vi "MOKE_Teperature and FIeld Sweep_1022D.vi"() -> ()   [LabVIEW 2022 SP3]
uses:
  <vilib>/Analysis/baseanly.llb/Mean (DBL).vi
  <vilib>/Utility/file.llb/Write Delimited Spreadsheet (string).vi
  <vilib>/Utility/file.llb/Write Delimited Spreadsheet (DBL).vi
  <vilib>/Analysis/NI_AALBase.lvlib
panel:
  in  "B field Drift Correction":bool
  in  "Scanner2 Drift Range (V)":dbl
  in  "Scanner1 Drift Range (V)":dbl
  in  "ANC300 address":refnum<visa-resource-name>="COM8"
  in  "Num Averages":i32=100
  in  "Read Status":bool
  in  "Wait for position/focus check every (Oe)":i32
  out "Rh1 B/A v F":cluster{dbl[], dbl[]}(graph)
  out "Temperature Status":i32(ring) items=["TemperatureUnknown"=0, "Stable"=1, "Tracking"=2, "Near"=5, "Chasing"=6, "Filling"=7, "Standby"=10, "Disabled"=13, "ImpedanceNotFunction"=14, "TempFailure"=15]
  out "Field Status":i32(ring) items=["MagnetUnknown"=0, "StablePersistent"=1, "WarmingSwitch"=2, "CoolingSwitch"=3, "StableDriven"=4, "Iterating"=5, "Charging"=6, "Discharging"=7, "CurrentError"=8, "MagnetFailure"=15]
  out "Field":dbl
  out "Temperature":dbl
  in  "Initialize":bool
  in  "System Stablization (s)":dbl=0.1 format="%#_13g"
  in  "Low Value (Oe)":dbl=-30000.0
  in  "High Value (Oe)":dbl=30000.0
  in  "Sweep Field Approach":i32(ring) items=["Linear", "NoOvershoot", "Oscillate"]
  in  "Sweep F Rate (Oe/s)":dbl=200.0 format="%#_13g"
  in  "Sweep F mode":i32(ring) items=["Persistent", "Driven"]
  in  "Set Fixed T":dbl=2.0
  in  "Fixed Temperature Approach":i32(ring)=1 items=["FastSettle", "NoOvershoot"]
  in  "FIxed T  Rate (K/min)":dbl=20.0
  out "PhaseA-F":cluster{dbl[], dbl[]}(graph)
  out "RA-F":cluster{dbl[], dbl[]}(graph)
  out "Phaseh1B-F":cluster{dbl[], dbl[]}(graph)
  out "Rh1B-F":cluster{dbl[], dbl[]}(graph)
  out "phase B 2":dbl
  in  "Phase B 2":u16(ring)=3 items=["X", "Y", "R", "Theta", "Frequency", "Noise", "Xh1", "Yh1", "Rh1", "Theta h1", "Xh2", "Yh2", "Rh2", "Theta h2"]
  out "phase A 2":dbl
  in  "Phase A 2":u16(ring)=3 items=["X", "Y", "R", "Theta", "Frequency", "Noise", "Xh1", "Yh1", "Rh1", "Theta h1", "Xh2", "Yh2", "Rh2", "Theta h2"]
  out "para1 Measurement (mV) 2":dbl=1.49013e-07
  in  "F Clear Plot A":bool
  in  "Parameter A 2":u16(ring)=2 items=["X", "Y", "R", "Theta", "Frequency", "Noise", "Xh1", "Yh1", "Rh1", "Theta h1", "Xh2", "Yh2", "Rh2", "Theta h2"]
  out "para2 Measurement (uV) 2":dbl=1.49013e-07
  in  "F Clear Plot B":bool
  in  "Parameter B 2":u16(ring)=2 items=["X", "Y", "R", "Theta", "Frequency", "Noise", "Xh1", "Yh1", "Rh1", "Theta h1", "Xh2", "Yh2", "Rh2", "Theta h2"]
  out "Field Setting":dbl format="%#_13g"
  out "Fixed Temperature":dbl
  out "Measured Field":dbl
  out "Field Status":i32(ring) items=["MagnetUnknown"=0, "StablePersistent"=1, "WarmingSwitch"=2, "CoolingSwitch"=3, "StableDriven"=4, "Iterating"=5, "Charging"=6, "Discharging"=7, "CurrentError"=8, "MagnetFailure"=15]
  out "Temperature Status":i32(ring) items=["TemperatureUnknown"=0, "Stable"=1, "Tracking"=2, "Near"=5, "Chasing"=6, "Filling"=7, "Standby"=10, "Disabled"=13, "ImpedanceNotFunction"=14, "TempFailure"=15]
  out "Measuring F":bool
  in  "Step(Oe)":i32=2000
  out "F loop run":i32
  out "Temperature Status":i32(ring) items=["TemperatureUnknown"=0, "Stable"=1, "Tracking"=2, "Near"=5, "Chasing"=6, "Filling"=7, "Standby"=10, "Disabled"=13, "ImpedanceNotFunction"=14, "TempFailure"=15]
  out "Field Status":i32(ring) items=["MagnetUnknown"=0, "StablePersistent"=1, "WarmingSwitch"=2, "CoolingSwitch"=3, "StableDriven"=4, "Iterating"=5, "Charging"=6, "Discharging"=7, "CurrentError"=8, "MagnetFailure"=15]
  out "Fixed Field":dbl
  out "Measured Temperature":dbl
  in  "Delay(T/F)":dbl=5.0
  in  "Set FIxed F (Oe)":dbl format="%#_13g"
  in  "Fixed Field Approach":i32(ring) items=["Linear", "NoOvershoot", "Oscillate"]
  in  "FIxed F Rate (Oe/s)":dbl=100.0 format="%#_13g"
  in  "Fixed F mode":i32(ring) items=["Persistent", "Driven"]
  in  "Sweep Temperature Approach":i32(ring)=1 items=["FastSettle", "NoOvershoot"]
  in  "Sweep T  Rate (K/min)":dbl=10.0
  in  "Sweep T/F":bool
  in  "Remote":bool=TRUE
  in  "IP Address":string="169.254.170.239"
  out "Measuring T":bool
  in  "A Sine Output Amplitude (V)":sgl=0.1
  in  "path (folder + filename)":string="C:\\Users\\Public\\OneDrive\\Desktop\\MOKE program\\sweep files"
  in  "LOCKIN address":refnum<visa-resource-name>="COM3"
  out "PhaseA-T":cluster{dbl[], dbl[]}(graph)
  out "RA-T":cluster{dbl[], dbl[]}(graph)
  out "Phaseh1-T":cluster{dbl[], dbl[]}(graph)
  out "Rh1B-T":cluster{dbl[], dbl[]}(graph)
  out "phase B":dbl
  in  "Phase B":u16(ring)=9 items=["X", "Y", "R", "Theta", "Frequency", "Noise", "Xh1", "Yh1", "Rh1", "Theta h1", "Xh2", "Yh2", "Rh2", "Theta h2"]
  out "phase A":dbl
  in  "Phase A":u16(ring)=3 items=["X", "Y", "R", "Theta", "Frequency", "Noise", "Xh1", "Yh1", "Rh1", "Theta h1", "Xh2", "Yh2", "Rh2", "Theta h2"]
  out "para1 Measurement (mV)":dbl=1.49013e-07
  in  "T Clear Plot A":bool
  in  "Parameter A":u16(ring)=2 items=["X", "Y", "R", "Theta", "Frequency", "Noise", "Xh1", "Yh1", "Rh1", "Theta h1", "Xh2", "Yh2", "Rh2", "Theta h2"]
  out "para2 Measurement (uV)":dbl=1.49013e-07
  in  "T Clear Plot B":bool
  in  "Parameter B":u16(ring)=8 items=["X", "Y", "R", "Theta", "Frequency", "Noise", "Xh1", "Yh1", "Rh1", "Theta h1", "Xh2", "Yh2", "Rh2", "Theta h2"]
  out "Temperature Setting":dbl format="%#_13g"
  in  "Save data or not":bool=TRUE
  in  "Step(K)":i32=10
  out "T loop run":i32
  in  "B frequency":dbl=267.7 format="%#_13g"
  in  "B Input Connection (0: Single-Ended)":u16(ring)=1 items=["Single-Ended Voltage", "Differential Voltage", "1 MOhm Current Gain", "100 MOhm Current Gain"]
  in  "B harmonic 1":u8=2
  in  "B harmonic 2":u8=3
  in  "B reference Manual Phase":dbl=-59.75
  in  "auto phase B":bool=TRUE
  in  "B Sample time (s)":dbl=0.001 min=0.001 max=100.0 step=0.001
  in  "B Sensitivity":u16(ring)=20 items=["1 nV/fA", "2 nV/fA", "5 nV/fA", "10 nV/fA", "20 nV/fA", "50 nV/fA", "100 nV/fA", "200 nV/fA", "500 nV/fA", "1 uV/pA", "2 uV/pA", "5 uV/pA", "10 uV/pA", "20 uV/pA", "50 uV/pA", "100 uV/pA", "200 uV/pA", "500 uV/pA", "1 mV/nA", "2 mV/nA", "5 mV/nA", "10 mV/nA", "20 mV/nA", "50 mV/nA", "100 mV/nA", "200 mV/nA", "500 mV/nA", "1 V/uA"]
  in  "Enable Sync Filter B (open when f<200Hz)":bool
  in  "B Time Constant":u8(ring)=9 items=["10 us", "30 us", "100 us", "300 us", "1 ms", "3 ms", "10 ms", "30 ms", "100 ms", "300 ms", "1 s", "3 s", "10 s", "30 s", "100 s", "300 s", "1 ks", "3 ks"]
  in  "B Reference Source":u8(ring) items=["External", "Internal", "Internal Sweep", "Channel-A"]
  in  "B Low Pass Filter Slope":u8(ring)=2 items=["6 dB/oct", "12 dB/oct", "18 db/oct", "24 dB/oct"]
  in  "A frequency":dbl=267.7 format="%#_13g"
  in  "A Input Connection (0: Single-Ended)":u16(ring)=1 items=["Single-Ended Voltage", "Differential Voltage", "1 MOhm Current Gain", "100 MOhm Current Gain"]
  in  "A harmonic 1":u8=2
  in  "A harmonic 2":u8=3
  in  "A reference Manual Phase":dbl=-59.75
  in  "auto phase A":bool=TRUE
  in  "A Reference Source":u8(ring) items=["External", "Internal", "Internal Sweep"]
  in  "A Sample time (s)":dbl=0.001 min=0.001 max=100.0 step=0.001
  in  "A Time Constant":u8(ring)=9 items=["10 us", "30 us", "100 us", "300 us", "1 ms", "3 ms", "10 ms", "30 ms", "100 ms", "300 ms", "1 s", "3 s", "10 s", "30 s", "100 s", "300 s", "1 ks", "3 ks"]
  in  "Enable Sync Filter A (open when f<200Hz)":bool
  in  "A Sensitivity":u16(ring)=20 items=["1 nV/fA", "2 nV/fA", "5 nV/fA", "10 nV/fA", "20 nV/fA", "50 nV/fA", "100 nV/fA", "200 nV/fA", "500 nV/fA", "1 uV/pA", "2 uV/pA", "5 uV/pA", "10 uV/pA", "20 uV/pA", "50 uV/pA", "100 uV/pA", "200 uV/pA", "500 uV/pA", "1 mV/nA", "2 mV/nA", "5 mV/nA", "10 mV/nA", "20 mV/nA", "50 mV/nA", "100 mV/nA", "200 mV/nA", "500 mV/nA", "1 V/uA"]
  in  "A Low Pass Filter Slope":u8(ring)=2 items=["6 dB/oct", "12 dB/oct", "18 db/oct", "24 dB/oct"]
  in  "stabilization(S)":dbl=0.1 format="%#_13g"
  in  "High Value (K)":dbl=300.0
  in  "Low Value (K)":dbl=2.0
  in  "loop #":i32=1
  # "Status"
  # "opticool ip addresse: 169.254.170.239"
  # "Lock-in Setting"
  # "Channel A"
  # "Channel B"
  # "Sweep F Mesurement"
  # "Temprature and Field Setting"
  # "Sweep T Mesurement"
  # "Sweep F"
  # "Sweep T"
  # "0 for no checks"
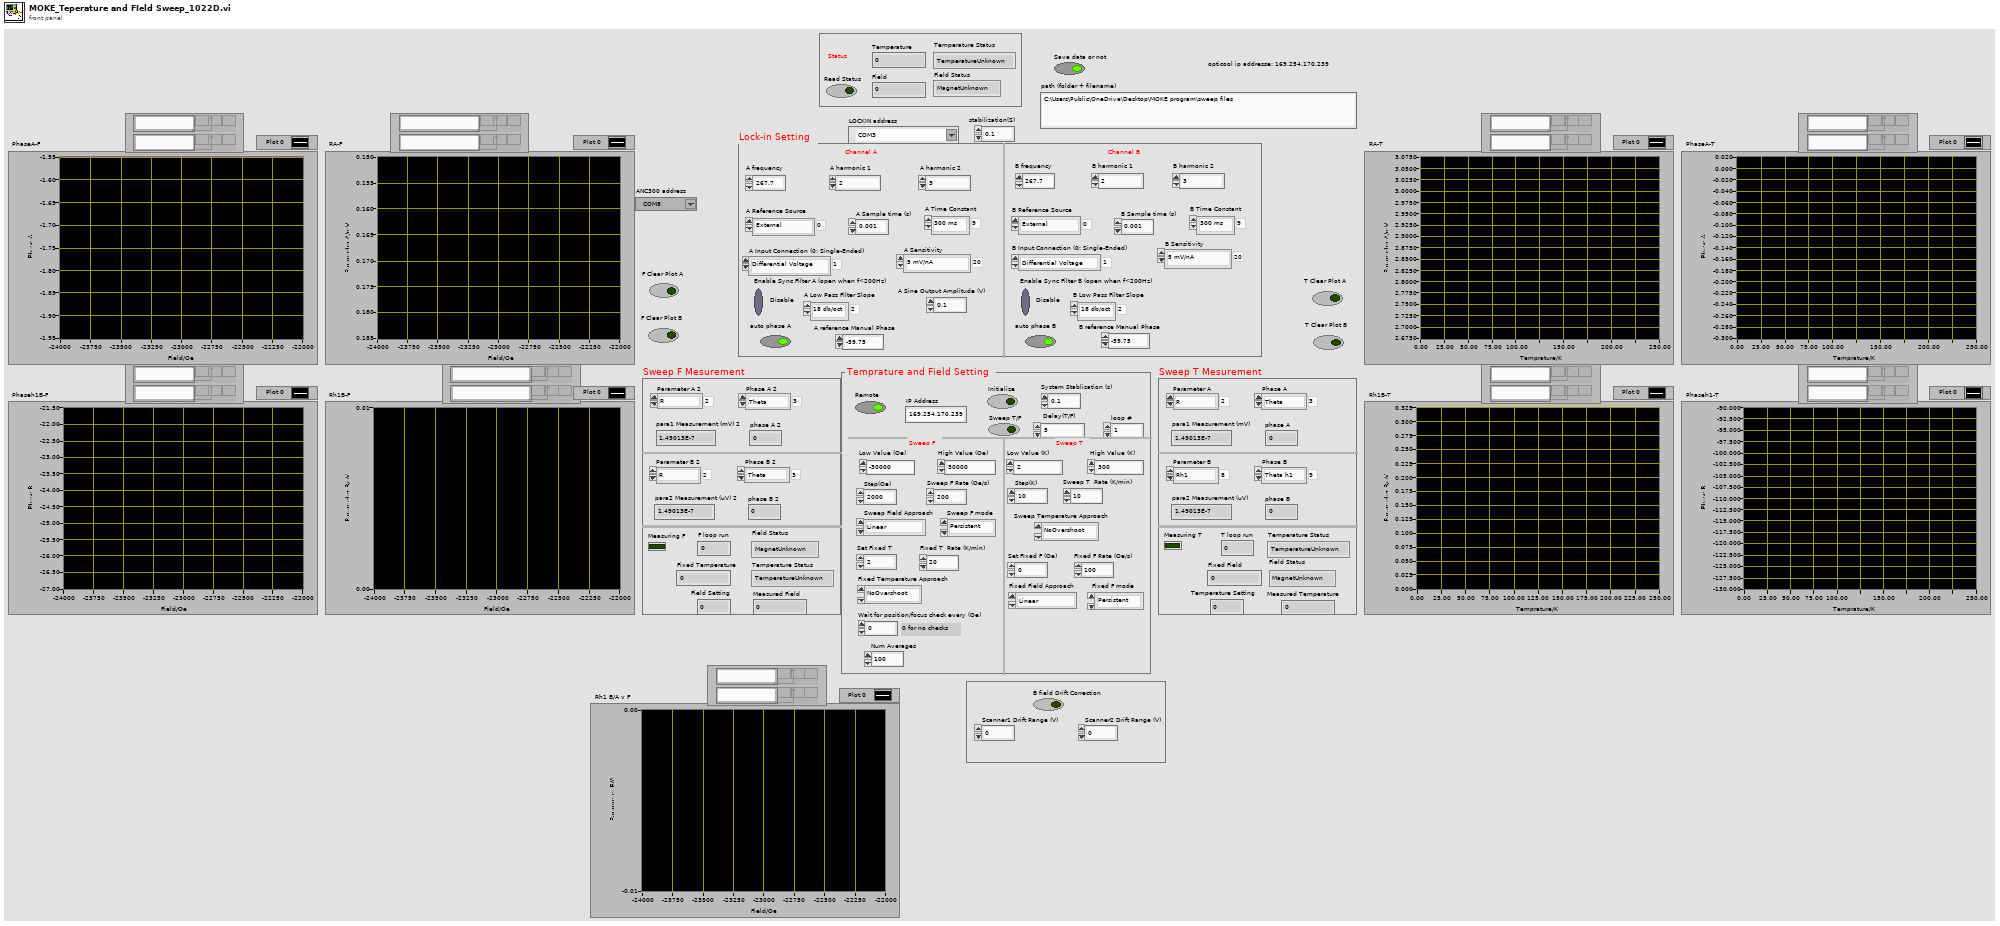
[diagram p1: front panel]
types:
  T1 = cluster{"error ":bool, "error number":i32, "error code":string}
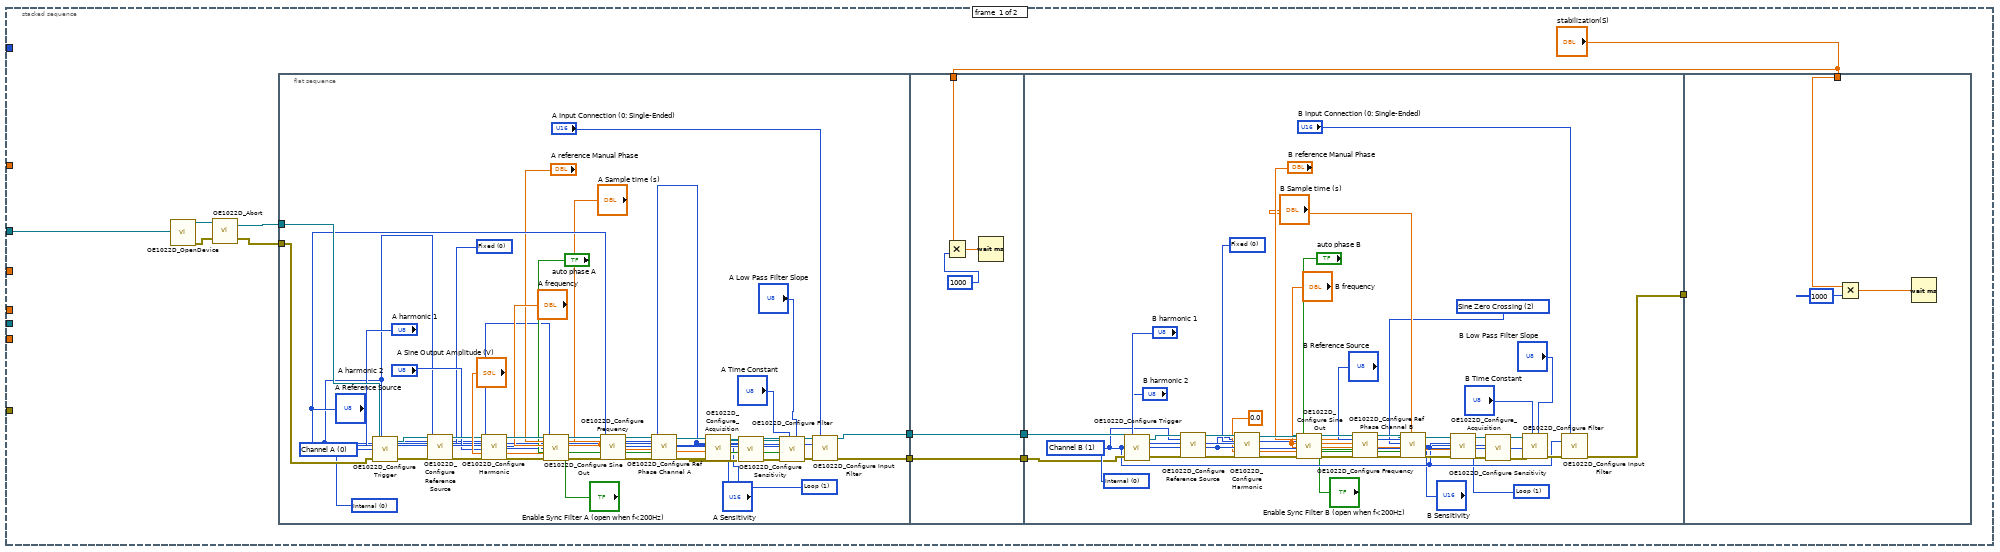
[diagram p3: hidden frame]
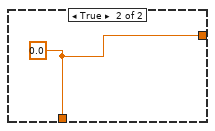
[diagram p5: hidden frame]
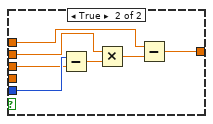
[diagram p9: hidden frame]
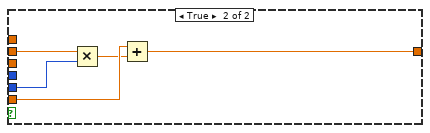
[diagram p10: hidden frame]
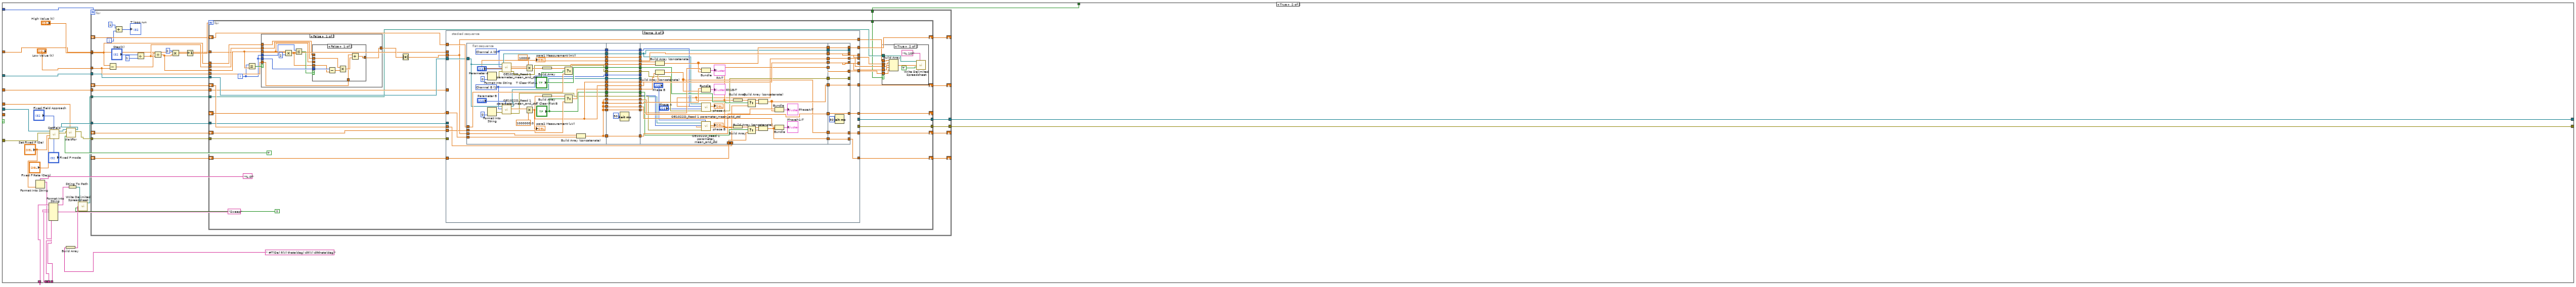
[diagram p11: hidden frame]
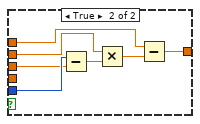
[diagram p13: hidden frame]
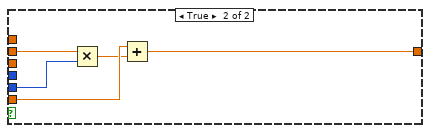
[diagram p14: hidden frame]
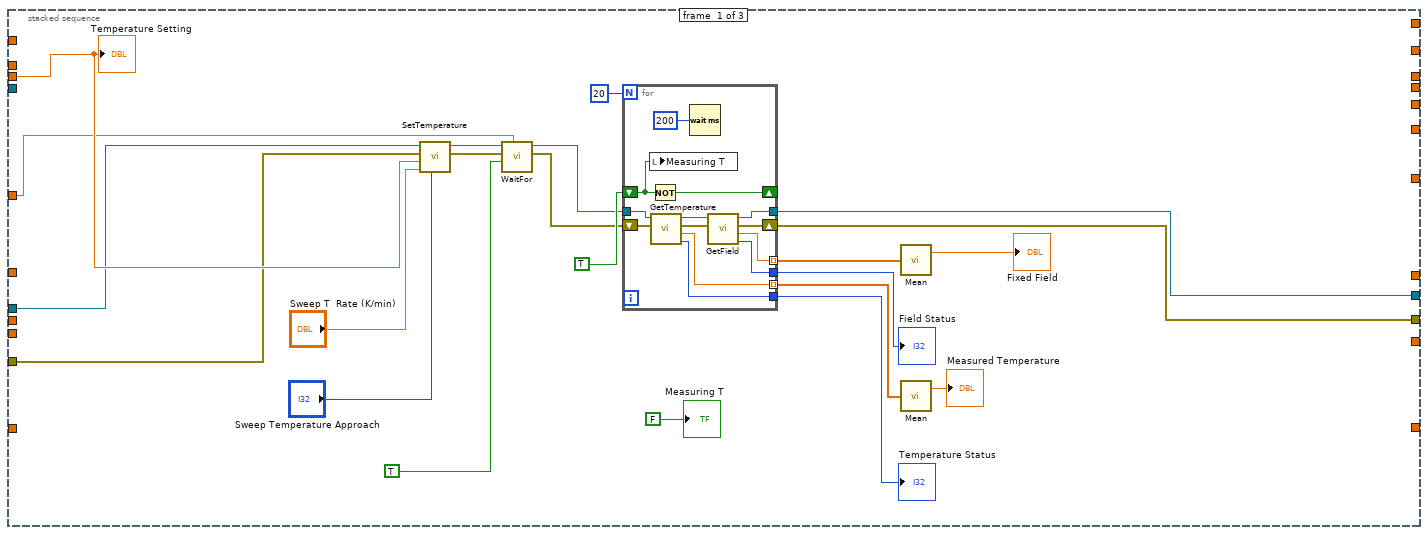
[diagram p15: hidden frame]
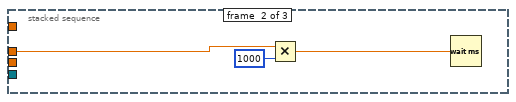
[diagram p16: hidden frame]
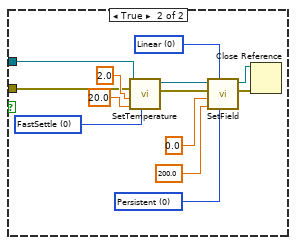
[diagram p17: hidden frame]
diagram:
  n1 = flat-sequence {
    tunnel: [w15] -> w13
    tunnel: [w14] -> w12
    tunnel: [w15] -> w5
    tunnel: [w14] -> w4
    tunnel: w13 -> [w29]
    tunnel: w12 -> [w28]
    tunnel: "path (folder + filename)" -> [w26]
    tunnel: "Oe" -> [w25]
    tunnel: "K" -> [w24]
    tunnel: ".txt" -> [w23]
    tunnel: [w21] -> w7
    tunnel: [w20] -> w6
    tunnel: "Save data or not" -> [w19]
    tunnel: w7 -> [w997]
    tunnel: w6 -> [w996]
    tunnel: [TRUE] -> w2
    frame #0 {
      w16 = 4 items=["PPMS", "VersaLab", "DynaCool", "SVSM", "OptiCool"] ("InstrumentType")
      n2 = call "OpenQDInstrument.vi"("Remote"="Remote", "IP Address"="IP Address", "InstrumentType"=w16) -> ("error out"=w14:errorcluster, "Instrument Ref"=w15:refnum<k24>)  [unwired: 5 in]
    }
    frame #1 {
      n3 = stacked-sequence {
        tunnel: "LOCKIN address" -> [w34 w143]
        tunnel: "loop #" -> [_ w142]
        tunnel: w29 -> [_ w140]
        tunnel: w28 -> [_ w139]
        tunnel: "Delay(T/F)" -> [_ w138]
        tunnel: "Delay(T/F)" -> [_ w137]
        tunnel: "Delay(T/F)" -> [_ w136]
        tunnel: w26 -> [_ w135]
        tunnel: w25 -> [_ w134]
        tunnel: w24 -> [_ w133]
        tunnel: w23 -> [_ w132]
        tunnel: "System Stablization (s)" -> [_ w131]
        tunnel: [_ w130] -> w21
        tunnel: [_ w129] -> w20
        tunnel: w19 -> [_ w128]
        frame #0 {
          n4 = call "OE1022D_OpenDevice.vi"("VISA resource name"=w34) -> ("VISA资源名称输出"=w33:refnum<visa-resource-name>, "错误输出"=w35:errorcluster)  [unwired: 17 in]
          n5 = call "OE1022D_Abort.vi"("error in (no error)"=w35, "VISA resource name"=w33) -> ("error out"=w40:errorcluster, "VISA resource name out"=w41:refnum<visa-resource-name>)
          n6 = flat-sequence {
            tunnel: w41 -> [w81]
            tunnel: [w69] -> w39
            tunnel: w40 -> [w80]
            tunnel: [w57] -> w37
            tunnel: w39 -> [w86]
            tunnel: [w86] -> w38
            tunnel: w37 -> [w85]
            tunnel: [w85] -> w36
            tunnel: "stabilization(S)" -> [w82]
            tunnel: w38 -> [w107]
            tunnel: [w106] -> w42
            tunnel: w36 -> [w105]
            tunnel: w42 -> [_]
            tunnel: "stabilization(S)" -> [w125]
            frame #0 {
              w43 = u8 1 items=["Single", "Loop"] ("Sample Mode (Single/Loop)")
              w56 = u8 0 items=["Fixed", "Linear", "Log"] ("SineOut Mode")
              w58 = u16 0 items=["Internal", "External"] ("Trigger Source (0: Internal)")
              w47 = u8 0 items=["Channel A", "Channel B"] ("OE1022D A/B")
              n7 = call "OE1022D_Configure Trigger.vi"("Trigger Source (0: Internal)"=w58, "error in (no error)   2"=w80, "OE1022D A/B"=w47, "VISA resource name   2"=w81) -> ("error out   2"=w74:errorcluster, "VISA resource name out   2"=w75:refnum<visa-resource-name>)
              n8 = call "OE1022D_Configure Reference Source.vi"("VISA resource name"=w75, "OE1022D A/B"=w47, "Reference Source"="A Reference Source", "error in (no error)"=w74) -> ("VISA resource name out"=w73:refnum<visa-resource-name>, "error out"=w71:errorcluster)  [unwired: 14 in]
              n9 = call "OE1022D_Configure Harmonic.vi"("VISA resource name"=w73, "OE1022D A/B"=w47, "Harmonic 1"="A harmonic 1", "Harmonic 2"="A harmonic 2", "error in (no error)"=w71) -> ("VISA resource name out"=w72:refnum<visa-resource-name>, "error out"=w70:errorcluster)  [unwired: 13 in]
              n10 = call "OE1022D_Configure Sine Out.vi"("VISA resource name"=w72, "SineOut Mode"=w56, "OE1022D A/B"=w47, "Sine Output Amplitude (V)"="A Sine Output Amplitude (V)", "error in (no error)"=w70) -> ("VISA resource name out"=w78:refnum<visa-resource-name>, "error out"=w77:errorcluster)  [unwired: 9 in]
              n11 = call "OE1022D_Configure Frequency.vi"("VISA resource name"=w78, "OE1022D A/B"=w47, "Internal Frequency(Hz)"="A frequency", "error in (no error)"=w77) -> ("VISA resource name out"=w68:refnum<visa-resource-name>, "error out"=w65:errorcluster)  [unwired: 14 in]
              n12 = call "OE1022D_Configure Ref Phase Channel A.vi"("VISA resource name"=w68, "Reference Source"="A Reference Source", "Internal Frequency(Hz)"="A frequency", "Auto Phase (T: Enabled)"="auto phase A", "error in (no error)"=w65, "Manual Phase  (degree)"="A reference Manual Phase") -> ("VISA resource name out"=w67:refnum<visa-resource-name>, "error out"=w66:errorcluster)  [unwired: 12 in]
              n13 = call "OE1022D_Configure_Acquisition.vi"("VISA resource name"=w67, "OE1022D A/B"=w47, "Sample time (s)"="A Sample time (s)", "error in (no error)"=w66, "Sample Mode (Single/Loop)"=w43) -> ("VISA resource name out"=w50:refnum<visa-resource-name>, "error out"=w49:errorcluster)  [unwired: 3 in]
              n14 = call "OE1022D_Configure Sensitivity.vi"("VISA resource name"=w50, "OE1022D A/B"=w47, "Sensitivity"="A Sensitivity", "error in (no error)"=w49) -> ("VISA resource name out"=w54:refnum<visa-resource-name>, "error out"=w53:errorcluster)  [unwired: 14 in]
              n15 = call "OE1022D_Configure Filter.vi"("Low Pass Filter Slope (1: 12dB/oct)"="A Low Pass Filter Slope", "Time Constant (8: 100ms)"="A Time Constant", "error in (no error)"=w53, "Enable Sync Filter (F: Disable)"="Enable Sync Filter A (open when f<200Hz)", "OE1022D A/B"=w47, "VISA resource name"=w54) -> ("error out"=w51:errorcluster, "VISA resource name out"=w52:refnum<visa-resource-name>)  [unwired: 4 in]
              n16 = call "OE1022D_Configure Input Filter.vi"("VISA resource name"=w52, "Input Source"="A Input Connection (0: Single-Ended)", "OE1022D A/B"=w47, "error in (no error)"=w51) -> ("VISA resource name out"=w57:refnum<visa-resource-name>, "error out"=w69:errorcluster)  [unwired: 10 in]
            }
            frame #1 {
              n17 = Multiply(x=w82, y=1000) -> (x*y=w84:dbl)
              n18 = Wait (ms)(milliseconds to wait=w84) -> ()  [unwired: 1 out]
            }
            frame #2 {
              w87 = u8 1 items=["Single", "Loop"] ("Sample Mode (Single/Loop)")
              w89 = u8 2 items=["TTL Pos", "TTL Neg", "Sine Zero Crossing"] ("External Ref Trigger")
              w102 = u8 0 items=["Fixed", "Linear", "Log"] ("SineOut Mode")
              w108 = u16 0 items=["Internal", "External"] ("Trigger Source (0: Internal)")
              w94 = u8 1 items=["Channel A", "Channel B"] ("OE1022D A/B")
              n19 = call "OE1022D_Configure Trigger.vi"("Trigger Source (0: Internal)"=w108, "error in (no error)   2"=w107, "OE1022D A/B"=w94, "VISA resource name   2"=w105) -> ("error out   2"=w120:errorcluster, "VISA resource name out   2"=w121:refnum<visa-resource-name>)
              n20 = call "OE1022D_Configure Reference Source.vi"("VISA resource name"=w121, "OE1022D A/B"=w94, "error in (no error)"=w120) -> ("VISA resource name out"=w119:refnum<visa-resource-name>, "error out"=w117:errorcluster)  [unwired: 15 in]
              n21 = call "OE1022D_Configure Harmonic.vi"("VISA resource name"=w119, "OE1022D A/B"=w94, "Harmonic 1"="B harmonic 1", "Harmonic 2"="B harmonic 2", "error in (no error)"=w117) -> ("VISA resource name out"=w118:refnum<visa-resource-name>, "error out"=w116:errorcluster)  [unwired: 13 in]
              n22 = call "OE1022D_Configure Sine Out.vi"("VISA resource name"=w118, "SineOut Mode"=w102, "OE1022D A/B"=w94, "Sine Output Amplitude (V)"=sgl 0.0, "error in (no error)"=w116) -> ("VISA resource name out"=w123:refnum<visa-resource-name>, "error out"=w122:errorcluster)  [unwired: 9 in]
              n23 = call "OE1022D_Configure Frequency.vi"("VISA resource name"=w123, "OE1022D A/B"=w94, "Internal Frequency(Hz)"="B frequency", "error in (no error)"=w122) -> ("VISA resource name out"=w115:refnum<visa-resource-name>, "error out"=w112:errorcluster)  [unwired: 14 in]
              n24 = call "OE1022D_Configure Ref Phase Channel B.vi"("VISA resource name"=w115, "Reference Source"="B Reference Source", "External Ref Trigger"=w89, "Internal Frequency(Hz)"="B frequency", "Auto Phase (T: Enabled)"="auto phase B", "error in (no error)"=w112, "Manual Phase  (degree)"="B reference Manual Phase") -> ("VISA resource name out"=w114:refnum<visa-resource-name>, "error out"=w113:errorcluster)  [unwired: 11 in]
              n25 = call "OE1022D_Configure_Acquisition.vi"("VISA resource name"=w114, "OE1022D A/B"=w94, "Sample time (s)"="B Sample time (s)", "error in (no error)"=w113, "Sample Mode (Single/Loop)"=w87) -> ("VISA resource name out"=w95:refnum<visa-resource-name>, "error out"=w96:errorcluster)  [unwired: 3 in]
              n26 = call "OE1022D_Configure Sensitivity.vi"("VISA resource name"=w95, "OE1022D A/B"=w94, "Sensitivity"="B Sensitivity", "error in (no error)"=w96) -> ("VISA resource name out"=w99:refnum<visa-resource-name>, "error out"=w98:errorcluster)  [unwired: 14 in]
              n27 = call "OE1022D_Configure Filter.vi"("Low Pass Filter Slope (1: 12dB/oct)"="B Low Pass Filter Slope", "Time Constant (8: 100ms)"="B Time Constant", "error in (no error)"=w98, "Enable Sync Filter (F: Disable)"="Enable Sync Filter B (open when f<200Hz)", "OE1022D A/B"=w94, "VISA resource name"=w99) -> ("error out"=w97:errorcluster)  [unwired: 4 in, 1 out]
              n28 = call "OE1022D_Configure Input Filter.vi"("Input Source"="B Input Connection (0: Single-Ended)", "OE1022D A/B"=w94, "error in (no error)"=w97) -> ("error out"=w106:errorcluster)  [unwired: 11 in, 1 out]
            }
            frame #3 {
              n29 = Multiply(x=w125, y=1000) -> (x*y=w127:dbl)
              n30 = Wait (ms)(milliseconds to wait=w127) -> ()  [unwired: 1 out]
            }
          }
        }
        frame #1 {
          n31 = case shown="False" "Sweep T/F" {
            tunnel: w143 -> [w175 w691]
            tunnel: w142 -> [w176 w690]
            tunnel: w140 -> [w167 w686]
            tunnel: w139 -> [w168 w685]
            tunnel: w138 -> [_ w679]
            tunnel: w137 -> [w174 w678]
            tunnel: w136 -> [w166 _]
            tunnel: w135 -> [w158 w674]
            tunnel: w134 -> [w157 w670]
            tunnel: w133 -> [w156 w671]
            tunnel: w132 -> [w155 w669]
            tunnel: w131 -> [w153 w666]
            tunnel: [w152 w665] -> w130
            tunnel: [w151 w664] -> w129
            tunnel: w128 -> [w150 w663]
            frame False {
              n32 = Format Into String(format string="%.1f", "Set Fixed T") -> (resulting string=w160:string)  [unwired: 2 in, 1 out]
              n33 = Format Into String(initial string=w158, w160, w156, "Sweep", w157, w155) -> (resulting string=w161:string)  [unwired: 2 in, 1 out]
              n34 = call "SetTemperature.vi"("Approach"="Fixed Temperature Approach", "Rate"="FIxed T  Rate (K/min)", "Temperature"="Set Fixed T", "error in (no error)"=w168, "Instrument Ref In"=w167) -> ("error out"=w169:errorcluster, "Instrument Ref Out"=w170:refnum<k24>)  [unwired: 2 in, 1 out]
              n35 = String To Path(string=w161) -> (path=w149:path)
              n36 = Build Array(" #B(Oe) R_mean(V) R_std(V) thetaR_mean(deg) thetaR_std(deg) dR_mean(V) dR_std(V) thetadR_mean(deg) thetadR_std(deg)") -> (w147:string[])
              n37 = call "WaitFor.vi"("Delay"=w166, "Wait For Temperature"=FALSE ("WaitForTemperature"), "error in (no error)"=w169, "Instrument Ref In"=w170) -> ("error out"=w165:errorcluster, "Instrument Ref Out"=w164:refnum<k24>)  [unwired: 6 in]
              n38 = call-poly <vilib>:"Write Delimited Spreadsheet.vi"("file path (dialog if empty)"=w149, "1D data"=w147, "append to file? (new file:F)"=TRUE) -> ("new file path (Not A Path if cancelled)"=w146:path)  [unwired: 11 in, 1 out]
              n39 = for {
                N: w176 -> [_]
                tunnel: w175 -> [w207]
                tunnel: "Low Value (Oe)" -> [w202]
                tunnel: "High Value (Oe)" -> [w192]
                tunnel: w146 -> [w201]
                shift-right: [w197] -> _
                shift-left: _ -> [w196]
                shift-right: [w191] -> _
                shift-left: _ -> [w190]
                shift-right: [w189] -> _
                shift-left: _ -> [w188]
                shift-right: [w187] -> _
                shift-left: _ -> [w186]
                tunnel: w164 -> [w185]
                tunnel: w165 -> [w184]
                tunnel: w174 -> [w183]
                tunnel: w153 -> [w182]
                shift-right: [w181] -> w152
                shift-left: _ -> [_]
                tunnel: [w180] -> w151
                tunnel: w150 -> [w179]
                tunnel: "Low Value (Oe)" -> [w177]
                i -> [w194]
                n40 = Subtract(x=w192, y=w202) -> (x-y=w204:dbl)
                n41 = Add(x=1, y=w194) -> (x+y=→"F loop run":i32)
                n42 = Divide(x="Step(Oe)", y=1) -> (x/y=w203:dbl)
                n43 = Divide(x=w204, y=w203) -> (x/y=w200:dbl)
                n44 = Multiply(x=2, y=w200) -> (x*y=w199:dbl)
                n45 = Increment(x=w199) -> (x+1=w198:dbl)
                n46 = for {
                  N: w198 -> [_]
                  tunnel: w207 -> [w272]
                  tunnel: w203 -> [w268]
                  shift-right: [w262] -> w197
                  shift-left: w196 -> [w271]
                  tunnel: w200 -> [w212]
                  tunnel: w202 -> [w269]
                  tunnel: w192 -> [w267]
                  tunnel: w201 -> [w247]
                  shift-right: [w261] -> _
                  shift-left: _ -> [w265]
                  shift-right: [w264] -> w191
                  shift-left: w190 -> [w263]
                  shift-right: [w260] -> w189
                  shift-left: w188 -> [w259]
                  shift-right: [w258] -> w187
                  shift-left: w186 -> [w257]
                  tunnel: w185 -> [w256]
                  tunnel: w184 -> [w255]
                  tunnel: w183 -> [w254]
                  tunnel: w182 -> [w253]
                  shift-right: [w252] -> w181
                  shift-left: _ -> [_]
                  tunnel: [w251] -> w180
                  tunnel: w179 -> [w250]
                  tunnel: "Step(Oe)" -> [w248]
                  shift-right: [w209] -> _
                  shift-left: w177 -> [w208]
                  i -> [w249]
                  n47 = Less Or Equal?(x=w249, y=w212) -> (x <= y?=w270:bool)
                  n48 = case shown="False" w270 {
                    tunnel: w269 -> [w629 w657]
                    tunnel: w249 -> [w638 w656]
                    tunnel: w268 -> [w637 w655]
                    tunnel: [w635 w653] -> w266
                    tunnel: w267 -> [w636 _]
                    tunnel: w212 -> [w631 _]
                    tunnel: w249 -> [w634 _]
                    frame False {
                      n49 = Multiply(x=w631, y=2) -> (x*y=w630:dbl)
                      n50 = Less Or Equal?(x=w634, y=w630) -> (x <= y?=w632:bool)
                      n51 = case shown="False" w632 {
                        tunnel: w638 -> [w645 w652]
                        tunnel: w637 -> [w643 w650]
                        tunnel: w636 -> [_ w648]
                        tunnel: [w641 w647] -> w635
                        tunnel: w631 -> [_ w646]
                        tunnel: w630 -> [w640 _]
                        tunnel: w629 -> [w639 _]
                        frame False {
                          n52 = Subtract(x=w645, y=w640) -> (x-y=w644:dbl)
                          n53 = Multiply(x=w643, y=w644) -> (x*y=w642:dbl)
                          n54 = Add(x=w639, y=w642) -> (x+y=w641:dbl)
                        }
                        frame True {
                          n55 = Subtract(x=w652, y=w646) -> (x-y=w651:dbl)
                          n56 = Multiply(x=w650, y=w651) -> (x*y=w649:dbl)
                          n57 = Subtract(x=w648, y=w649) -> (x-y=w647:dbl)
                        }
                      }
                    }
                    frame True {
                      n58 = Multiply(x=w655, y=w656) -> (x*y=w654:dbl)
                      n59 = Add(x=w657, y=w654) -> (x+y=w653:dbl)
                    }
                  }
                  n60 = flat-sequence {
                    tunnel: w272 -> [w288]
                    tunnel: [w288] -> w236
                    tunnel: w266 -> [w290]
                    tunnel: [w290] -> w235
                    tunnel: w271 -> [w287]
                    tunnel: [w287] -> w234
                    tunnel: w265 -> [w286]
                    tunnel: [w286] -> w233
                    tunnel: w263 -> [w285]
                    tunnel: [w285] -> w232
                    tunnel: w259 -> [w284]
                    tunnel: [w284] -> w231
                    tunnel: w257 -> [w283]
                    tunnel: [w283] -> w230
                    tunnel: w256 -> [w295]
                    tunnel: w255 -> [w294]
                    tunnel: w254 -> [w293]
                    tunnel: w253 -> [w282]
                    tunnel: [w282] -> w229
                    tunnel: [w292] -> w228
                    tunnel: [w291] -> w227
                    tunnel: w249 -> [w281]
                    tunnel: [w281] -> w226
                    tunnel: w248 -> [w280]
                    tunnel: [w280] -> w225
                    tunnel: w208 -> [w289]
                    tunnel: [w275] -> w224
                    tunnel: [w279] -> w213
                    tunnel: w212 -> [w277]
                    tunnel: [w278] -> w211
                    tunnel: [w273] -> w210
                    tunnel: w236 -> [w344]
                    tunnel: [w344] -> w223
                    tunnel: w235 -> [w343]
                    tunnel: [w343] -> w222
                    tunnel: w234 -> [w342]
                    tunnel: [w342] -> w221
                    tunnel: w233 -> [w341]
                    tunnel: [w341] -> w220
                    tunnel: w232 -> [w340]
                    tunnel: [w340] -> w219
                    tunnel: w231 -> [w339]
                    tunnel: [w339] -> w218
                    tunnel: w230 -> [w338]
                    tunnel: [w338] -> w217
                    tunnel: w229 -> [w354]
                    tunnel: w228 -> [w337]
                    tunnel: [w337] -> w216
                    tunnel: w227 -> [w336]
                    tunnel: [w336] -> w215
                    tunnel: w226 -> [w353]
                    tunnel: w225 -> [w352]
                    tunnel: w224 -> [w335]
                    tunnel: [w335] -> w214
                    tunnel: w213 -> [w334]
                    tunnel: w211 -> [w327]
                    tunnel: w210 -> [w326]
                    tunnel: w223 -> [w497]
                    tunnel: w222 -> [w496]
                    tunnel: w221 -> [w499]
                    tunnel: [w498] -> w262
                    tunnel: [w484] -> w246
                    tunnel: [w496] -> w244
                    tunnel: [w495] -> w261
                    tunnel: w220 -> [w494]
                    tunnel: [w493] -> w241
                    tunnel: [w492] -> w264
                    tunnel: w219 -> [w485]
                    tunnel: [w491] -> w260
                    tunnel: w218 -> [w486]
                    tunnel: [w490] -> w258
                    tunnel: w217 -> [w489]
                    tunnel: [w488] -> w242
                    tunnel: [w487] -> w243
                    tunnel: [w418] -> w252
                    tunnel: w216 -> [w418]
                    tunnel: [w417] -> w251
                    tunnel: w215 -> [w417]
                    tunnel: [w429] -> w240
                    tunnel: [w425] -> w239
                    tunnel: [w423] -> w238
                    tunnel: [w421] -> w237
                    tunnel: [w416] -> w209
                    tunnel: w214 -> [w416]
                    frame #0 {
                      n61 = Divide(x=w277, y=2) -> (x/y=w278:dbl)
                      n62 = call "SetField.vi"("Mode"="Sweep F mode", "Approach"="Sweep Field Approach", "Rate"="Sweep F Rate (Oe/s)", "Field"=w290, "error in (no error)"=w294, "Instrument Ref In"=w295) -> ("error out"=w299:errorcluster, "Instrument Ref Out"=w300:refnum<k24>)  [unwired: 1 in, 1 out]
                      n63 = call "WaitFor.vi"("Delay"=w293, "Wait For Field"=TRUE, "error in (no error)"=w299, "Instrument Ref In"=w300) -> ("error out"=w297:errorcluster, "Instrument Ref Out"=w296:refnum<k24>)  [unwired: 6 in]
                      n64 = for {
                        N: 5 -> [_]
                        shift-right: [w325] -> _
                        shift-left: TRUE -> [w323]
                        shift-right: [w320] -> w292
                        shift-left: w297 -> [w322]
                        tunnel: w296 -> [w319]
                        tunnel: [w317] -> w291
                        tunnel: [w314] -> w310
                        tunnel: [w313] -> w309
                        tunnel: [w315] -> w307 mode=indexing
                        tunnel: [w316] -> w308 mode=indexing
                        n65 = local write "Measuring F"(w323) -> ()
                        n66 = Not(x=w323) -> (.not. x?=w325:bool)
                        n67 = call "GetTemperature.vi"("error in (no error)"=w322, "Instrument Ref In"=w319) -> ("Temperature\nStatus"=w313:i32, "Temperature"=w316:dbl, "error out"=w321:errorcluster, "Instrument Ref Out"=w318:refnum<k24>)  [unwired: 3 in, 1 out]
                        n68 = Wait (ms)(milliseconds to wait=u32 100) -> ()  [unwired: 1 out]
                        n69 = call "GetField.vi"("error in (no error)"=w321, "Instrument Ref In"=w318) -> ("Field\nStatus"=w314:i32, "Field"=w315:dbl, "error out"=w320:errorcluster, "Instrument Ref Out"=w317:refnum<k24>)  [unwired: 3 in, 1 out]
                      }
                      "Field Status" <- w310
                      "Temperature Status" <- w309
                      n70 = call-poly <vilib>:"Mean.vi"("X"=w307) -> ("mean"=→"Measured Field":dbl)  [unwired: 1 out]
                      n71 = call-poly <vilib>:"Mean.vi"("X"=w308) -> ("mean"=→"Fixed Temperature":dbl)  [unwired: 1 out]
                      n72 = Absolute Value(x=w289) -> (abs(x)=w274:dbl)
                      n73 = Absolute Value(x=w290) -> (abs(x)=w275:dbl)
                      n74 = Equal?(x=w275, y=w274) -> (x = y?=w273:bool)
                      n75 = Less?(x=w275, y=w274) -> (x < y?=w279:bool)
                      "Field Setting" <- w290
                      "Measuring F" <- FALSE
                    }
                    frame #1 {
                      # "this is where we could add a drift correction automatically"
                      n76 = Multiply(x=w353, y=w352) -> (x*y=w351:i32)
                      n77 = Quotient & Remainder(x=w351, y="Wait for position/focus check every (Oe)") -> (x-y*floor(x/y)=w350:i32)  [unwired: 1 out]
                      n78 = Divide(x="Scanner1 Drift Range (V)", y=w327) -> (x/y=w329:dbl)
                      n79 = Divide(x="Scanner2 Drift Range (V)", y=w327) -> (x/y=w330:dbl)
                      n80 = Not Equal To 0?(x="Wait for position/focus check every (Oe)") -> (x != 0?=w346:bool)
                      n81 = Equal To 0?(x=w350) -> (x = 0?=w349:bool)
                      n82 = case shown="False" w326 {
                        tunnel: w334 -> [w361 _]
                        tunnel: [w360 w369] -> w333
                        tunnel: [w359 w369] -> w332
                        tunnel: w330 -> [w358 _]
                        tunnel: w329 -> [w357 _]
                        frame False {
                          n83 = case shown="True" w361 {
                            tunnel: w357 -> [w362 w367]
                            tunnel: w358 -> [w363 w368]
                            tunnel: [w362 w366] -> w360
                            tunnel: [w363 w365] -> w359
                            frame False {
                            }
                            frame True {
                              w364 = -1.0
                              n84 = Multiply(x=w364, y=w368) -> (x*y=w365:dbl)
                              n85 = Multiply(x=w367, y=w364) -> (x*y=w366:dbl)
                            }
                          }
                        }
                        frame True {
                          w369 = 0.0
                        }
                      }
                      n86 = Multiply(x=w354, y=1000) -> (x*y=w356:dbl)
                      n87 = case shown="True" "B field Drift Correction" {
                        tunnel: w333 -> [_ w379]
                        tunnel: w332 -> [_ w376]
                        frame False {
                        }
                        frame True {
                          w386 = 2
                          w387 = 1
                          w389 = "a "  # Voltage
                          w385 = FALSE  # set / get
                          w393 = "a "  # Voltage
                          w399 = 2
                          w400 = 1
                          w401 = TRUE  # set / get
                          w403 = "a "  # Voltage
                          w406 = TRUE  # set / get
                          w408 = "a "  # Voltage
                          w396 = u32 100 ("millisecond timer value")
                          n88 = call "ANC300_Open.vi"("ANC300 Communication Port In"="ANC300 address", "milliseconds to wait"=w396) -> ("ANC300 Communication Port Out"=w411:refnum<visa-resource-name>, "error out"=w412:T1)  [unwired: 13 in, 3 out]
                          n89 = call "ANC300_GetSerial.vi"("ANC300 Communication Port In"=w411, "error in"=w412) -> ("ANC300 Communication Port Out"=w384:refnum<visa-resource-name>, "error out"=w383:T1)  [unwired: 10 in, 6 out]
                          n90 = call "ANC300_Mode.vi"("ANC300 Communication Port In"=w384, "Axis"=w387, "axis mode in"="off", "error in"=w383, "set / get"=w385) -> ("ANC300 Communication Port Out"=w395:refnum<visa-resource-name>, "error out"=w394:T1)  [unwired: 8 in, 5 out]
                          n91 = call "ANC300_Preferences.vi"("ANC300 Communication Port In"=w395, "Axis"=w387, "parameter"=w393, "error in"=w394, "set / get"=w385) -> ("ANC300 Communication Port Out"=w373:refnum<visa-resource-name>, "value out"=w380:dbl, "error out"=w382:T1)  [unwired: 7 in, 5 out]
                          n92 = call "ANC300_Mode.vi"("ANC300 Communication Port In"=w373, "Axis"=w386, "axis mode in"="off", "error in"=w382, "set / get"=w385) -> ("ANC300 Communication Port Out"=w391:refnum<visa-resource-name>, "error out"=w390:T1)  [unwired: 8 in, 5 out]
                          n93 = call "ANC300_Preferences.vi"("ANC300 Communication Port In"=w391, "Axis"=w386, "parameter"=w389, "error in"=w390, "set / get"=w385) -> ("ANC300 Communication Port Out"=w375:refnum<visa-resource-name>, "value out"=w381:dbl, "error out"=w374:T1)  [unwired: 7 in, 5 out]
                          n94 = Add(x=w381, y=w376) -> (x+y=w377:dbl)
                          n95 = Add(x=w380, y=w379) -> (x+y=w378:dbl)
                          n96 = call "ANC300_Mode.vi"("ANC300 Communication Port In"=w375, "Axis"=w400, "axis mode in"="off", "error in"=w374, "set / get"=w406) -> ("ANC300 Communication Port Out"=w410:refnum<visa-resource-name>, "error out"=w409:T1)  [unwired: 8 in, 5 out]
                          n97 = call "ANC300_Preferences.vi"("ANC300 Communication Port In"=w410, "Axis"=w400, "value in"=w378, "parameter"=w408, "error in"=w409, "set / get"=w406) -> ("ANC300 Communication Port Out"=w397:refnum<visa-resource-name>, "error out"=w398:T1)  [unwired: 6 in, 6 out]
                          n98 = Wait (ms)(milliseconds to wait=w396) -> ()  [unwired: 1 out]
                          n99 = call "ANC300_Mode.vi"("ANC300 Communication Port In"=w397, "Axis"=w399, "axis mode in"="off", "error in"=w398, "set / get"=w401) -> ("ANC300 Communication Port Out"=w405:refnum<visa-resource-name>, "error out"=w404:T1)  [unwired: 8 in, 5 out]
                          n100 = call "ANC300_Preferences.vi"("ANC300 Communication Port In"=w405, "Axis"=w399, "value in"=w377, "parameter"=w403, "error in"=w404, "set / get"=w401) -> ("ANC300 Communication Port Out"=w370:refnum<visa-resource-name>, "error out"=w371:T1)  [unwired: 6 in, 6 out]
                          n101 = Wait (ms)(milliseconds to wait=1500) -> ()  [unwired: 1 out]
                          n102 = call "ANC300_Close.vi"("ANC300 Communication Port In"=w370, "error in"=w371) -> ()  [unwired: 17 in, 1 out]
                        }
                      }
                      n103 = And(x=w349, y=w346) -> (x .and. y?=w348:bool)
                      n104 = flat-sequence {
                        tunnel: w356 -> [w414]
                        tunnel: w348 -> [w415]
                        frame #0 {
                          n105 = Wait (ms)(milliseconds to wait=w414) -> ()  [unwired: 1 out]
                        }
                        frame #1 {
                          n106 = case shown="True" w415 {
                            frame False {
                            }
                            frame True {
                              n107 = call "Prompt User for Input"() -> ()  [unwired: 17 in, 3 out]
                            }
                          }
                        }
                      }
                    }
                    frame #2 {
                      n108 = flat-sequence {
                        tunnel: w499 -> [w532]
                        tunnel: w497 -> [w505]
                        tunnel: w496 -> [w531]
                        tunnel: w494 -> [w530]
                        tunnel: w489 -> [w527]
                        tunnel: [w510] -> w483
                        tunnel: [w520] -> w482
                        tunnel: [w522] -> w481
                        tunnel: [w521] -> w480
                        tunnel: [w522] -> w479
                        tunnel: [w522] -> w478
                        tunnel: [w522] -> w477
                        tunnel: [w522] -> w476
                        tunnel: [w520] -> w475
                        tunnel: [w526] -> w474
                        tunnel: [w521] -> w473
                        tunnel: [w525] -> w472
                        tunnel: ["F Clear Plot B"] -> w471
                        tunnel: ["F Clear Plot A"] -> w470
                        tunnel: [w515] -> w469
                        tunnel: [w518] -> w468
                        tunnel: [w514] -> w467
                        tunnel: [w509] -> w466
                        tunnel: [w506] -> w465
                        tunnel: [w522] -> w464
                        tunnel: [w502] -> w430
                        tunnel: [w501] -> w426
                        tunnel: ["Num Averages"] -> w419
                        tunnel: w483 -> [w558]
                        tunnel: [w558] -> w463
                        tunnel: w482 -> [w557]
                        tunnel: [w557] -> w462
                        tunnel: w481 -> [w556]
                        tunnel: [w556] -> w461
                        tunnel: w480 -> [w555]
                        tunnel: [w555] -> w460
                        tunnel: w479 -> [w554]
                        tunnel: [w554] -> w459
                        tunnel: w478 -> [w553]
                        tunnel: [w553] -> w458
                        tunnel: w477 -> [w552]
                        tunnel: [w552] -> w457
                        tunnel: w476 -> [w551]
                        tunnel: [w551] -> w456
                        tunnel: w475 -> [w550]
                        tunnel: [w550] -> w455
                        tunnel: w474 -> [w549]
                        tunnel: [w549] -> w454
                        tunnel: w473 -> [w548]
                        tunnel: [w548] -> w453
                        tunnel: w472 -> [w547]
                        tunnel: [w547] -> w452
                        tunnel: w471 -> [w546]
                        tunnel: [w546] -> w451
                        tunnel: w470 -> [w545]
                        tunnel: [w545] -> w450
                        tunnel: w469 -> [w544]
                        tunnel: [w544] -> w449
                        tunnel: w468 -> [w543]
                        tunnel: [w543] -> w448
                        tunnel: w467 -> [w542]
                        tunnel: [w542] -> w447
                        tunnel: w466 -> [w541]
                        tunnel: [w541] -> w446
                        tunnel: w465 -> [w540]
                        tunnel: [w540] -> w445
                        tunnel: [w538] -> w444
                        tunnel: w464 -> [w538]
                        tunnel: [w537] -> w431
                        tunnel: w430 -> [w537]
                        tunnel: [w536] -> w427
                        tunnel: w426 -> [w536]
                        tunnel: [w535] -> w420
                        tunnel: w419 -> [w535]
                        tunnel: w463 -> [w567]
                        tunnel: w462 -> [w608]
                        tunnel: w461 -> [w607]
                        tunnel: w460 -> [w606]
                        tunnel: w459 -> [w605]
                        tunnel: w458 -> [w585]
                        tunnel: w457 -> [w584]
                        tunnel: w456 -> [w601]
                        tunnel: w455 -> [w598]
                        tunnel: w454 -> [w597]
                        tunnel: w453 -> [w595]
                        tunnel: w452 -> [w594]
                        tunnel: w486 -> [w593]
                        tunnel: w451 -> [w592]
                        tunnel: w485 -> [w590]
                        tunnel: w450 -> [w589]
                        tunnel: w449 -> [w568]
                        tunnel: w448 -> [w569]
                        tunnel: w447 -> [w570]
                        tunnel: w446 -> [w564]
                        tunnel: w445 -> [w566]
                        tunnel: [w567] -> w443
                        tunnel: [w583] -> w442
                        tunnel: [w608] -> w441
                        tunnel: [w607] -> w440
                        tunnel: [w562] -> w439
                        tunnel: [w563] -> w438
                        tunnel: [w599] -> w437
                        tunnel: [w596] -> w436
                        tunnel: [w582] -> w435
                        tunnel: [w606] -> w434
                        tunnel: [w572] -> w433
                        tunnel: w444 -> [w581]
                        tunnel: [w574] -> w432
                        tunnel: w431 -> [w574]
                        tunnel: [w573] -> w428
                        tunnel: w427 -> [w573]
                        tunnel: [w561] -> w424
                        tunnel: [w560] -> w422
                        tunnel: w420 -> [w559]
                        tunnel: [w614] -> w487
                        tunnel: [w615] -> w488
                        tunnel: [w616] -> w490
                        tunnel: [w617] -> w491
                        tunnel: [w618] -> w492
                        tunnel: [w619] -> _
                        tunnel: [w620] -> w493
                        tunnel: [w621] -> w495
                        tunnel: [w622] -> w484
                        tunnel: [w623] -> w498
                        tunnel: [w624] -> _
                        tunnel: w443 -> [w624]
                        tunnel: w442 -> [w623]
                        tunnel: w441 -> [w622]
                        tunnel: w440 -> [w621]
                        tunnel: w439 -> [w620]
                        tunnel: w438 -> [w619]
                        tunnel: w437 -> [w618]
                        tunnel: w436 -> [w617]
                        tunnel: w435 -> [w616]
                        tunnel: w434 -> [w615]
                        tunnel: w433 -> [w614]
                        tunnel: [w612] -> w429
                        tunnel: w432 -> [w612]
                        tunnel: [w611] -> w425
                        tunnel: w428 -> [w611]
                        tunnel: [w610] -> w423
                        tunnel: w424 -> [w610]
                        tunnel: w422 -> [w609]
                        tunnel: [w609] -> w421
                        frame #0 {
                          w503 = 1.0 ("y")
                          w512 = 1.0 ("y")
                          w518 = u8 1 items=["Channel A", "Channel B"] ("Channel A/B for Parameter1")
                          w506 = u8 0 items=["Channel A", "Channel B"] ("Channel A/B for Parameter1")
                          n109 = Format Into String(0) -> (error out=w519:errorcluster)  [unwired: 3 in, 1 out]
                          n110 = Format Into String(0) -> (error out=w508:errorcluster)  [unwired: 3 in, 1 out]
                          n111 = call "OE1022D_Read 1 parameter_mean_and_std.vi"("Num Averages"="Num Averages", "Parameter 2"="Parameter B 2", "错误输入（无错误）"=w519, "Channel (0: A)"=w518, "VISA resource name"=w505) -> ("error out"=w515:errorcluster, "Measurement"=w516:dbl, "VISA resource name out"=w514:refnum<visa-resource-name>, "Measurement STD"=w513:dbl)  [unwired: 3 in]
                          n112 = call "OE1022D_Read 1 parameter_mean_and_std.vi"("错误输入（无错误）"=w508, "Parameter"="Parameter A 2", "Channel (0: A)"=w506, "VISA resource name"=w505) -> ("error out"=w509:errorcluster, "Measurement"=w511:dbl, "VISA resource name out"=w510:refnum<visa-resource-name>, "Measurement STD"=w504:dbl)  [unwired: 4 in]
                          n113 = Multiply(x=w516, y=w512) -> (x*y=w521:dbl)
                          "para2 Measurement (uV) 2" <- w521
                          n114 = Multiply(x=w511, y=w503) -> (x*y=w520:dbl)
                          "para1 Measurement (mV) 2" <- w520
                          n115 = Multiply(x=w504, y=w503) -> (x*y=w502:dbl)
                          n116 = Build Array(w520) -> (w533:dbl[])
                          n117 = Build Array(w521) -> (w528:dbl[])
                          n118 = Select(t=w528, s="F Clear Plot B", f=w527) -> (s? t:f=w525:dbl[])
                          n119 = Select(t=w533, s="F Clear Plot A", f=w532) -> (s? t:f=w526:dbl[])
                          n120 = Build Array (concatenate)(w531, w530) -> (w522:dbl[])
                          n121 = Multiply(x=w513, y=w512) -> (x*y=w501:dbl)
                        }
                        frame #1 {
                          n122 = Wait (ms)(milliseconds to wait=u32 50) -> ()  [unwired: 1 out]
                        }
                        frame #2 {
                          n123 = Build Array (concatenate)(w598, w597) -> (w583:dbl[])
                          n124 = Build Array (concatenate)(w595, w594) -> (w582:dbl[])
                          n125 = call "OE1022D_Read 1 parameter_mean_and_std.vi"("Num Averages"=w559, "Parameter 2"="Phase B 2", "错误输入（无错误）"=w568, "Channel (0: A)"=w569, "VISA resource name"=w570) -> ("Measurement"=w572:dbl, "Measurement STD"=w561:dbl)  [unwired: 3 in, 2 out]
                          "phase B 2" <- w572
                          n126 = Bundle(w584, w583) -> (→"RA-F":cluster{dbl[], dbl[]})  [unwired: 1 in]
                          n127 = Bundle(w585, w582) -> (→"Rh1B-F":cluster{dbl[], dbl[]})  [unwired: 1 in]
                          n128 = call "OE1022D_Read 1 parameter_mean_and_std.vi"("Num Averages"=w559, "错误输入（无错误）"=w564, "Parameter"="Phase A 2", "Channel (0: A)"=w566, "VISA resource name"=w567) -> ("error out"=w563:errorcluster, "Measurement"=w562:dbl, "Measurement STD"=w560:dbl)  [unwired: 3 in, 1 out]
                          "phase A 2" <- w562
                          n129 = Divide(x=w582, y=w583) -> (x/y=w577:dbl[])
                          n130 = Build Array(w562) -> (w586:dbl[])
                          n131 = Build Array(w572) -> (w587:dbl[])
                          n132 = Select(t=w586, s=w589, f=w590) -> (s? t:f=w588:dbl[])
                          n133 = Select(t=w587, s=w592, f=w593) -> (s? t:f=w591:dbl[])
                          n134 = Sign(1:w572) -> (0:w575:dbl)
                          n135 = Negate(x=w577) -> (-x=w578:dbl[])
                          n136 = Build Array (concatenate)(w562, w588) -> (w599:dbl[])
                          n137 = Build Array (concatenate)(w572, w591) -> (w596:dbl[])
                          n138 = Greater Or Equal To 0?(x=w575) -> (x >= 0?=w576:bool)
                          n139 = Select(t=w577, s=w576, f=w578) -> (s? t:f=w579:dbl[])
                          n140 = Bundle(w601, w599) -> (→"PhaseA-F":cluster{dbl[], dbl[]})  [unwired: 1 in]
                          n141 = Bundle(w605, w596) -> (→"Phaseh1B-F":cluster{dbl[], dbl[]})  [unwired: 1 in]
                          n142 = Bundle(w581, w579) -> (→"Rh1 B/A v F":cluster{dbl[], dbl[]})  [unwired: 1 in]
                        }
                        frame #3 {
                          n143 = Wait (ms)(milliseconds to wait=u32 50) -> ()  [unwired: 1 out]
                        }
                      }
                    }
                  }
                  n144 = Build Array(w244, w246, w240, w241, w237, w242, w239, w243, w238) -> (w245:dbl[])
                  n145 = case shown="True" w250 {
                    tunnel: w247 -> [_ w625]
                    tunnel: w245 -> [_ w628]
                    frame False {
                    }
                    frame True {
                      n146 = call-poly <vilib>:"Write Delimited Spreadsheet.vi"("file path (dialog if empty)"=w625, "format (%.3f)"="%.10f", "1D data"=w628, "append to file? (new file:F)"=TRUE) -> ()  [unwired: 10 in, 2 out]
                    }
                  }
                }
              }
            }
            frame True {
              n147 = Format Into String(format string="%.0f", "Set FIxed F (Oe)") -> (resulting string=w673:string)  [unwired: 2 in, 1 out]
              n148 = Format Into String(initial string=w674, "Sweep", w671, w673, w670, w669) -> (resulting string=w675:string)  [unwired: 2 in, 1 out]
              n149 = call "SetField.vi"("Mode"="Fixed F mode", "Approach"="Fixed Field Approach", "Rate"="FIxed F Rate (Oe/s)", "Field"="Set FIxed F (Oe)", "error in (no error)"=w685, "Instrument Ref In"=w686) -> ("error out"=w681:errorcluster, "Instrument Ref Out"=w683:refnum<k24>)  [unwired: 1 in, 1 out]
              n150 = Build Array(" #T(Oe) R(V) theta(deg) dR(V) dRtheta(deg)") -> (w662:string[])
              n151 = call "WaitFor.vi"("Delay"=w679, "Wait For Field"=TRUE, "error in (no error)"=w681, "Instrument Ref In"=w683) -> ("error out"=w682:errorcluster, "Instrument Ref Out"=w684:refnum<k24>)  [unwired: 6 in]
              n152 = String To Path(string=w675) -> (path=w659:path)
              n153 = call-poly <vilib>:"Write Delimited Spreadsheet.vi"("file path (dialog if empty)"=w659, "1D data"=w662, "append to file? (new file:F)"=TRUE) -> ("new file path (Not A Path if cancelled)"=w658:path)  [unwired: 11 in, 1 out]
              n154 = for {
                N: w690 -> [_]
                tunnel: w691 -> [w721]
                tunnel: "Low Value (K)" -> [w715]
                tunnel: "High Value (K)" -> [w705]
                tunnel: w658 -> [w714]
                shift-right: [w710] -> _
                shift-left: _ -> [w709]
                shift-right: [w704] -> _
                shift-left: _ -> [w703]
                shift-right: [w702] -> _
                shift-left: _ -> [w701]
                shift-right: [w700] -> _
                shift-left: _ -> [w699]
                tunnel: w684 -> [w698]
                tunnel: w682 -> [w697]
                tunnel: w678 -> [w696]
                tunnel: w666 -> [w695]
                tunnel: [w694] -> w665
                tunnel: [w693] -> w664
                tunnel: w663 -> [w692]
                i -> [w707]
                n155 = Subtract(x=w705, y=w715) -> (x-y=w717:dbl)
                n156 = Add(x=1, y=w707) -> (x+y=→"T loop run":i32)
                n157 = Divide(x="Step(K)", y=1) -> (x/y=w716:dbl)
                n158 = Divide(x=w717, y=w716) -> (x/y=w713:dbl)
                n159 = Multiply(x=2, y=w713) -> (x*y=w712:dbl)
                n160 = Increment(x=w712) -> (x+1=w711:dbl)
                n161 = for {
                  N: w711 -> [_]
                  tunnel: w721 -> [w753]
                  tunnel: w716 -> [w749]
                  shift-right: [w740] -> w710
                  shift-left: w709 -> [w752]
                  tunnel: w713 -> [w747]
                  tunnel: w715 -> [w750]
                  tunnel: w705 -> [w748]
                  tunnel: w714 -> [w724]
                  shift-right: [w729] -> _
                  shift-left: _ -> [w743]
                  shift-right: [w742] -> w704
                  shift-left: w703 -> [w741]
                  shift-right: [w739] -> w702
                  shift-left: w701 -> [w738]
                  shift-right: [w737] -> w700
                  shift-left: w699 -> [w736]
                  tunnel: w698 -> [w735]
                  tunnel: w697 -> [w734]
                  tunnel: w696 -> [w733]
                  tunnel: w695 -> [w732]
                  tunnel: [w731] -> w694
                  tunnel: [w730] -> w693
                  tunnel: w692 -> [w722]
                  i -> [w746]
                  n162 = Less Or Equal?(x=w746, y=w747) -> (x <= y?=w751:bool)
                  n163 = case shown="False" w751 {
                    tunnel: w750 -> [w763 w791]
                    tunnel: w746 -> [w772 w790]
                    tunnel: w749 -> [w771 w789]
                    tunnel: [w769 w787] -> w745
                    tunnel: w748 -> [w770 _]
                    tunnel: w747 -> [w765 _]
                    tunnel: w746 -> [w768 _]
                    frame False {
                      n164 = Multiply(x=w765, y=2) -> (x*y=w764:dbl)
                      n165 = Less Or Equal?(x=w768, y=w764) -> (x <= y?=w766:bool)
                      n166 = case shown="False" w766 {
                        tunnel: w772 -> [w779 w786]
                        tunnel: w771 -> [w777 w784]
                        tunnel: w770 -> [_ w782]
                        tunnel: [w775 w781] -> w769
                        tunnel: w765 -> [_ w780]
                        tunnel: w764 -> [w774 _]
                        tunnel: w763 -> [w773 _]
                        frame False {
                          n167 = Subtract(x=w779, y=w774) -> (x-y=w778:dbl)
                          n168 = Multiply(x=w777, y=w778) -> (x*y=w776:dbl)
                          n169 = Add(x=w773, y=w776) -> (x+y=w775:dbl)
                        }
                        frame True {
                          n170 = Subtract(x=w786, y=w780) -> (x-y=w785:dbl)
                          n171 = Multiply(x=w784, y=w785) -> (x*y=w783:dbl)
                          n172 = Subtract(x=w782, y=w783) -> (x-y=w781:dbl)
                        }
                      }
                    }
                    frame True {
                      n173 = Multiply(x=w789, y=w790) -> (x*y=w788:dbl)
                      n174 = Add(x=w791, y=w788) -> (x+y=w787:dbl)
                    }
                  }
                  n175 = Absolute Value(x=w745) -> (abs(x)=w744:dbl)
                  n176 = stacked-sequence {
                    tunnel: w753 -> [_ _ w892]
                    tunnel: w744 -> [w810 _ w830]
                    tunnel: w752 -> [_ _ w894]
                    tunnel: [_ _ w893] -> w740
                    tunnel: [_ _ w891] -> w725
                    tunnel: [_ _ w890] -> w729
                    tunnel: w743 -> [_ _ w889]
                    tunnel: [_ _ w888] -> w726
                    tunnel: [_ _ w887] -> w742
                    tunnel: w741 -> [_ _ w881]
                    tunnel: [_ _ w886] -> w739
                    tunnel: w738 -> [_ _ w882]
                    tunnel: [_ _ w885] -> w737
                    tunnel: w736 -> [_ _ w884]
                    tunnel: [_ _ w831] -> w727
                    tunnel: [_ _ w883] -> w728
                    tunnel: w735 -> [w809 _ _]
                    tunnel: w734 -> [w808 _ _]
                    tunnel: w733 -> [w805 _ _]
                    tunnel: w732 -> [_ w827 _]
                    tunnel: [w793 _ _] -> w731
                    tunnel: [w792 _ _] -> w730
                    tunnel: [_ _ w830] -> w723
                    frame #0 {
                      n177 = call "SetTemperature.vi"("Approach"="Sweep Temperature Approach", "Rate"="Sweep T  Rate (K/min)", "Temperature"=w810, "error in (no error)"=w808, "Instrument Ref In"=w809) -> ("error out"=w806:errorcluster, "Instrument Ref Out"=w807:refnum<k24>)  [unwired: 2 in, 1 out]
                      n178 = call "WaitFor.vi"("Delay"=w805, "Wait For Temperature"=TRUE ("WaitForTemperature"), "error in (no error)"=w806, "Instrument Ref In"=w807) -> ("error out"=w796:errorcluster, "Instrument Ref Out"=w795:refnum<k24>)  [unwired: 6 in]
                      n179 = for {
                        N: 20 -> [_]
                        shift-right: [w826] -> _
                        shift-left: TRUE -> [w824]
                        shift-right: [w821] -> w793
                        shift-left: w796 -> [w823]
                        tunnel: w795 -> [w820]
                        tunnel: [w818] -> w792
                        tunnel: [w815] -> w802
                        tunnel: [w814] -> w801
                        tunnel: [w816] -> w799 mode=indexing
                        tunnel: [w817] -> w800 mode=indexing
                        n180 = local write "Measuring T"(w824) -> ()
                        n181 = Not(x=w824) -> (.not. x?=w826:bool)
                        n182 = call "GetTemperature.vi"("error in (no error)"=w823, "Instrument Ref In"=w820) -> ("Temperature\nStatus"=w814:i32, "Temperature"=w817:dbl, "error out"=w822:errorcluster, "Instrument Ref Out"=w819:refnum<k24>)  [unwired: 3 in, 1 out]
                        n183 = Wait (ms)(milliseconds to wait=u32 200) -> ()  [unwired: 1 out]
                        n184 = call "GetField.vi"("error in (no error)"=w822, "Instrument Ref In"=w819) -> ("Field\nStatus"=w815:i32, "Field"=w816:dbl, "error out"=w821:errorcluster, "Instrument Ref Out"=w818:refnum<k24>)  [unwired: 3 in, 1 out]
                      }
                      "Field Status" <- w802
                      "Temperature Status" <- w801
                      n185 = call-poly <vilib>:"Mean.vi"("X"=w799) -> ("mean"=→"Fixed Field":dbl)  [unwired: 1 out]
                      n186 = call-poly <vilib>:"Mean.vi"("X"=w800) -> ("mean"=→"Measured Temperature":dbl)  [unwired: 1 out]
                      "Temperature Setting" <- w810
                      "Measuring T" <- FALSE
                    }
                    frame #1 {
                      n187 = Multiply(x=w827, y=1000) -> (x*y=w829:dbl)
                      n188 = Wait (ms)(milliseconds to wait=w829) -> ()  [unwired: 1 out]
                    }
                    frame #2 {
                      n189 = flat-sequence {
                        tunnel: w894 -> [w922]
                        tunnel: w892 -> [w913]
                        tunnel: w830 -> [w921]
                        tunnel: w889 -> [w920]
                        tunnel: w884 -> [w911]
                        tunnel: [w918] -> w880
                        tunnel: [w905] -> w878
                        tunnel: [w906] -> w876
                        tunnel: [w903] -> w874
                        tunnel: [w906] -> w872
                        tunnel: [w906] -> w870
                        tunnel: [w906] -> w868
                        tunnel: [w906] -> w866
                        tunnel: [w905] -> w864
                        tunnel: [w904] -> w862
                        tunnel: [w903] -> w860
                        tunnel: [w902] -> w858
                        tunnel: ["T Clear Plot B"] -> w856
                        tunnel: ["T Clear Plot A"] -> w854
                        tunnel: [w899] -> w852
                        tunnel: [w898] -> w850
                        tunnel: [w897] -> w848
                        tunnel: [w896] -> w846
                        tunnel: [w895] -> w844
                        tunnel: w880 -> [w944]
                        tunnel: [w944] -> w879
                        tunnel: w878 -> [w943]
                        tunnel: [w943] -> w877
                        tunnel: w876 -> [w942]
                        tunnel: [w942] -> w875
                        tunnel: w874 -> [w941]
                        tunnel: [w941] -> w873
                        tunnel: w872 -> [w940]
                        tunnel: [w940] -> w871
                        tunnel: w870 -> [w939]
                        tunnel: [w939] -> w869
                        tunnel: w868 -> [w938]
                        tunnel: [w938] -> w867
                        tunnel: w866 -> [w937]
                        tunnel: [w937] -> w865
                        tunnel: w864 -> [w936]
                        tunnel: [w936] -> w863
                        tunnel: w862 -> [w935]
                        tunnel: [w935] -> w861
                        tunnel: w860 -> [w934]
                        tunnel: [w934] -> w859
                        tunnel: w858 -> [w933]
                        tunnel: [w933] -> w857
                        tunnel: w856 -> [w932]
                        tunnel: [w932] -> w855
                        tunnel: w854 -> [w931]
                        tunnel: [w931] -> w853
                        tunnel: w852 -> [w930]
                        tunnel: [w930] -> w851
                        tunnel: w850 -> [w929]
                        tunnel: [w929] -> w849
                        tunnel: w848 -> [w928]
                        tunnel: [w928] -> w847
                        tunnel: w846 -> [w927]
                        tunnel: [w927] -> w845
                        tunnel: w844 -> [w926]
                        tunnel: [w926] -> w843
                        tunnel: w879 -> [w948]
                        tunnel: w877 -> [w982]
                        tunnel: w875 -> [w981]
                        tunnel: w873 -> [w980]
                        tunnel: w871 -> [w979]
                        tunnel: w869 -> [w977]
                        tunnel: w867 -> [w975]
                        tunnel: w865 -> [w973]
                        tunnel: w863 -> [w970]
                        tunnel: w861 -> [w969]
                        tunnel: w859 -> [w966]
                        tunnel: w857 -> [w965]
                        tunnel: w882 -> [w963]
                        tunnel: w855 -> [w962]
                        tunnel: w881 -> [w960]
                        tunnel: w853 -> [w959]
                        tunnel: w851 -> [w955]
                        tunnel: w849 -> [w954]
                        tunnel: w847 -> [w953]
                        tunnel: w845 -> [w950]
                        tunnel: w843 -> [w949]
                        tunnel: [w948] -> w842
                        tunnel: [w968] -> w841
                        tunnel: [w982] -> w840
                        tunnel: [w981] -> w839
                        tunnel: [w946] -> w838
                        tunnel: [w947] -> w837
                        tunnel: [w971] -> w836
                        tunnel: [w967] -> w835
                        tunnel: [w964] -> w834
                        tunnel: [w980] -> w833
                        tunnel: [w952] -> w832
                        tunnel: [w986] -> w883
                        tunnel: [w987] -> w831
                        tunnel: [w984] -> w885
                        tunnel: [w988] -> w886
                        tunnel: [w989] -> w887
                        tunnel: [w990] -> _
                        tunnel: [w991] -> w888
                        tunnel: [w992] -> w890
                        tunnel: [w993] -> w891
                        tunnel: [w983] -> w893
                        tunnel: [w994] -> _
                        tunnel: w842 -> [w994]
                        tunnel: w841 -> [w983]
                        tunnel: w840 -> [w993]
                        tunnel: w839 -> [w992]
                        tunnel: w838 -> [w991]
                        tunnel: w837 -> [w990]
                        tunnel: w836 -> [w989]
                        tunnel: w835 -> [w988]
                        tunnel: w834 -> [w984]
                        tunnel: w833 -> [w987]
                        tunnel: w832 -> [w986]
                        frame #0 {
                          w898 = u8 1 items=["Channel A", "Channel B"] ("Channel A/B for Parameter1")
                          w895 = u8 0 items=["Channel A", "Channel B"] ("Channel A/B for Parameter1")
                          n190 = Format Into String(0) -> (error out=w919:errorcluster)  [unwired: 3 in, 1 out]
                          n191 = Format Into String(0) -> (error out=w914:errorcluster)  [unwired: 3 in, 1 out]
                          n192 = call "OE1022D_Read 1 parameter_mean_and_std.vi"("错误输入（无错误）"=w919, "Parameter"="Parameter A", "Channel (0: A)"=w895, "VISA resource name"=w913) -> ("error out"=w896:errorcluster, "Measurement"=w908:dbl, "VISA resource name out"=w918:refnum<visa-resource-name>)  [unwired: 4 in, 1 out]
                          n193 = call "OE1022D_Read 1 parameter_mean_and_std.vi"("Parameter 2"="Parameter B", "错误输入（无错误）"=w914, "Channel (0: A)"=w898, "VISA resource name"=w913) -> ("error out"=w899:errorcluster, "Measurement"=w907:dbl, "VISA resource name out"=w897:refnum<visa-resource-name>)  [unwired: 4 in, 1 out]
                          n194 = Multiply(x=w908, y=1000.0) -> (x*y=w905:dbl)
                          "para1 Measurement (mV)" <- w905
                          n195 = Multiply(x=w907, y=1000000.0) -> (x*y=w903:dbl)
                          "para2 Measurement (uV)" <- w903
                          n196 = Build Array(w905) -> (w923:dbl[])
                          n197 = Build Array(w903) -> (w915:dbl[])
                          n198 = Select(t=w923, s="T Clear Plot A", f=w922) -> (s? t:f=w904:dbl[])
                          n199 = Select(t=w915, s="T Clear Plot B", f=w911) -> (s? t:f=w902:dbl[])
                          n200 = Build Array (concatenate)(w921, w920) -> (w906:dbl[])
                        }
                        frame #1 {
                          n201 = Wait (ms)(milliseconds to wait=u32 50) -> ()  [unwired: 1 out]
                        }
                        frame #2 {
                          n202 = Build Array (concatenate)(w970, w969) -> (w968:dbl[])
                          n203 = Build Array (concatenate)(w966, w965) -> (w964:dbl[])
                          n204 = Bundle(w975, w968) -> (→"RA-T":cluster{dbl[], dbl[]})  [unwired: 1 in]
                          n205 = Bundle(w977, w964) -> (→"Rh1B-T":cluster{dbl[], dbl[]})  [unwired: 1 in]
                          n206 = call "OE1022D_Read 1 parameter_mean_and_std.vi"("错误输入（无错误）"=w950, "Parameter"="Phase A", "Channel (0: A)"=w949, "VISA resource name"=w948) -> ("error out"=w947:errorcluster, "Measurement"=w946:dbl)  [unwired: 4 in, 2 out]
                          "phase A" <- w946
                          n207 = call "OE1022D_Read 1 parameter_mean_and_std.vi"("Parameter 2"="Phase B", "错误输入（无错误）"=w955, "Channel (0: A)"=w954, "VISA resource name"=w953) -> ("Measurement"=w952:dbl)  [unwired: 4 in, 3 out]
                          "phase B" <- w952
                          n208 = Build Array(w946) -> (w956:dbl[])
                          n209 = Build Array(w952) -> (w957:dbl[])
                          n210 = Select(t=w956, s=w959, f=w960) -> (s? t:f=w958:dbl[])
                          n211 = Select(t=w957, s=w962, f=w963) -> (s? t:f=w961:dbl[])
                          n212 = Build Array (concatenate)(w946, w958) -> (w971:dbl[])
                          n213 = Build Array (concatenate)(w952, w961) -> (w967:dbl[])
                          n214 = Bundle(w973, w971) -> (→"PhaseA-T":cluster{dbl[], dbl[]})  [unwired: 1 in]
                          n215 = Bundle(w979, w967) -> (→"Phaseh1-T":cluster{dbl[], dbl[]})  [unwired: 1 in]
                        }
                        frame #3 {
                          n216 = Wait (ms)(milliseconds to wait=u32 50) -> ()  [unwired: 1 out]
                        }
                      }
                    }
                  }
                  n217 = case shown="True" w722 {
                    tunnel: w725 -> [_ w757]
                    tunnel: w723 -> [_ w762]
                    tunnel: w724 -> [_ w760]
                    tunnel: w726 -> [_ w756]
                    tunnel: w727 -> [_ w755]
                    tunnel: w728 -> [_ w754]
                    frame False {
                    }
                    frame True {
                      n218 = Build Array(w762, w757, w756, w755, w754) -> (w759:dbl[])
                      n219 = call-poly <vilib>:"Write Delimited Spreadsheet.vi"("file path (dialog if empty)"=w760, "format (%.3f)"="%.10f", "1D data"=w759, "append to file? (new file:F)"=TRUE) -> ()  [unwired: 10 in, 2 out]
                    }
                  }
                }
              }
            }
          }
        }
      }
    }
    frame #2 {
      n220 = case shown="False" "Initialize" {
        tunnel: w997 -> [w998 w1001]
        tunnel: w996 -> [w999 w1000]
        frame False {
          n221 = Close Reference(reference=w999, error in (no error)=w998) -> ()  [unwired: 1 out]
        }
        frame True {
          w1007 = 0 items=["Linear", "NoOvershoot", "Oscillate"] ("Approach")
          w1008 = 0 items=["Persistent", "Driven"] ("Mode")
          w1004 = 0 items=["FastSettle", "NoOvershoot"] ("Approach")
          n222 = call "SetTemperature.vi"("Approach"=w1004, "Rate"=20.0, "Temperature"=2.0, "error in (no error)"=w1001, "Instrument Ref In"=w1000) -> ("error out"=w1012:errorcluster, "Instrument Ref Out"=w1011:refnum<k24>)  [unwired: 2 in, 1 out]
          n223 = call "SetField.vi"("Mode"=w1008, "Approach"=w1007, "Rate"=200.0, "Field"=0.0, "error in (no error)"=w1012, "Instrument Ref In"=w1011) -> ("error out"=w1009:errorcluster, "Instrument Ref Out"=w1010:refnum<k24>)  [unwired: 1 in, 1 out]
          n224 = Close Reference(reference=w1010, error in (no error)=w1009) -> ()  [unwired: 1 out]
        }
      }
    }
    frame #3 {
    }
  }
  n225 = case shown="True" "Read Status" {
    tunnel: w5 -> [_ w1016]
    tunnel: w4 -> [_ w1015]
    tunnel: w2 -> [_ w1014]
    frame False {
    }
    frame True {
      n226 = while {
        tunnel: w1016 -> [w1019]
        tunnel: w1015 -> [w1018]
        tunnel: w1014 -> [w1017]
        stop <- w1017 stop-if-true
        n227 = for {
          N: 10 -> [_]
          shift-right: [w1034] -> _
          shift-left: w1018 -> [w1036]
          tunnel: w1019 -> [w1033]
          tunnel: [w1031] -> _
          tunnel: [w1028] -> w1025
          tunnel: [w1027] -> w1024
          tunnel: [w1029] -> w1022 mode=indexing
          tunnel: [w1030] -> w1023 mode=indexing
          n228 = call "GetTemperature.vi"("error in (no error)"=w1036, "Instrument Ref In"=w1033) -> ("Temperature\nStatus"=w1027:i32, "Temperature"=w1030:dbl, "error out"=w1035:errorcluster, "Instrument Ref Out"=w1032:refnum<k24>)  [unwired: 3 in, 1 out]
          n229 = Wait (ms)(milliseconds to wait=u32 200) -> ()  [unwired: 1 out]
          n230 = call "GetField.vi"("error in (no error)"=w1035, "Instrument Ref In"=w1032) -> ("Field\nStatus"=w1028:i32, "Field"=w1029:dbl, "error out"=w1034:errorcluster, "Instrument Ref Out"=w1031:refnum<k24>)  [unwired: 3 in, 1 out]
        }
        "Field Status" <- w1025
        "Temperature Status" <- w1024
        n231 = call-poly <vilib>:"Mean.vi"("X"=w1022) -> ("mean"=→"Field":dbl)  [unwired: 1 out]
        n232 = call-poly <vilib>:"Mean.vi"("X"=w1023) -> ("mean"=→"Temperature":dbl)  [unwired: 1 out]
      }
    }
  }
